vi "test3-SafeStr conversion.vi"(8 "error in (no error)":errorcluster, 11 "TestCase in":refnum<class "testcase-CSMArgument.lvclass">) -> (0 "error out":errorcluster, 3 "TestCase out":refnum<class "testcase-CSMArgument.lvclass">)   [LabVIEW 2017, in "testcase-CSMArgument.lvclass"]
uses:
  testcase-CSMArgument.lvclass
  src/user.lib/_NEVSTOP/Communicable State Machine(CSM)/AdvanceAPI/CSM - Keywords.vi
  <vilib>/addons/_JKI Toolkits/VI Tester/TestCase.llb/TestCase.lvclass
  src/user.lib/_NEVSTOP/Communicable State Machine(CSM)/Communicable State Machine.lvlib
  C:/Program Files (x86)/National Instruments/LabVIEW 2017/vi.lib/addons/_JKI Toolkits/VI Tester/TestCase.llb/TestCase.lvclass
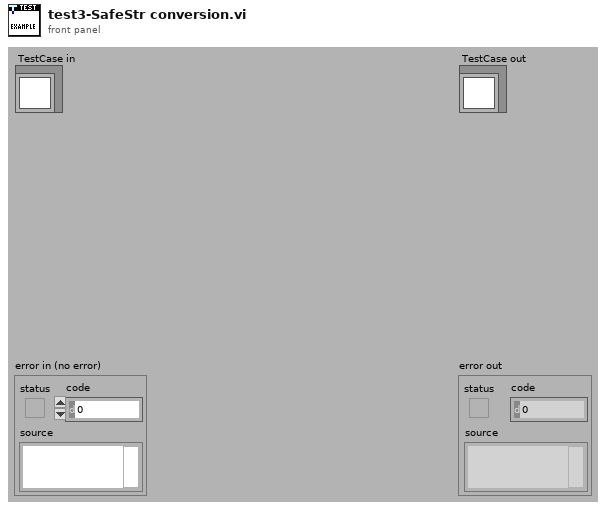
[diagram p1: front panel]
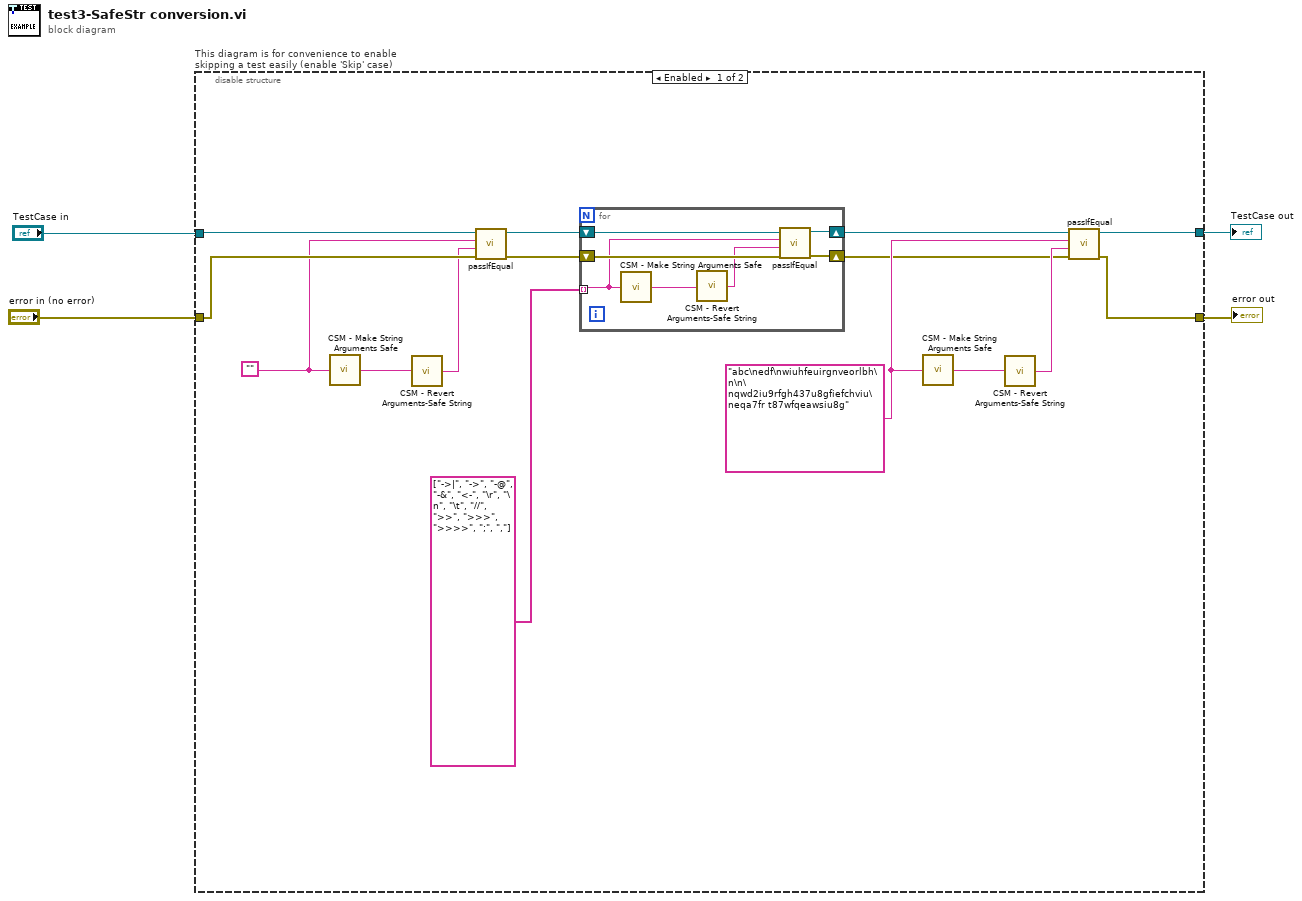
[diagram p0: block diagram]
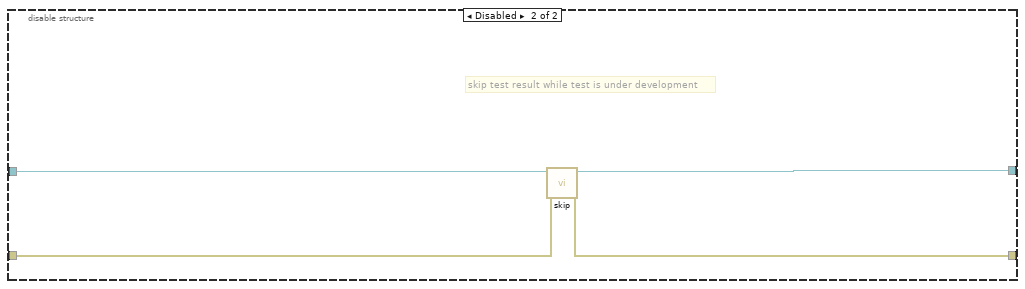
[diagram p2: hidden frame]
diagram:
  n1 = disable-structure "This diagram is for convenience to enable skipping a test easily (enable 'Skip' case)" shown="Enabled" {
    disable-tunnel: "TestCase in" -> [w19 w30]
    disable-tunnel: [w8 w28] -> w1
    disable-tunnel: [w6 w29] -> w3
    disable-tunnel: "error in (no error)" -> [w18 w27]
    frame Enabled {
      w10 = "abc\nedf\nwiuhfeuirgnveorlbh\n\n\nqwd2iu9rfgh437u8gfiefchviu\neqa7fr t87wfqeawsiu8g"
      w16 = ""
      n2 = call "CSM - Make String Arguments Safe.vi"("Argument String"=w16) -> ("Safe Argument String"=w17:string)  [unwired: 8 in]
      n3 = call "CSM - Revert Arguments-Safe String.vi"("Safe Argument String"=w17) -> ("Origin Argument String"=w15:string)  [unwired: 8 in]
      n4 = call-dynamic "passIfEqual.vi"("error in (no error)"=w18, "y"=w15, "x"=w16, "TestCase in"=w19) -> ("error out"=w12:errorcluster, "TestCase out"=w13:refnum<class "testcase-CSMArgument.lvclass">)  [unwired: 6 in]
      n5 = for {
        tunnel: string[] ["->|", "->", "-@", "-&", "<-", "\r", "\n", "\t", "//", ">>", ">>>", ">>>>", ";", ","] -> [w21] mode=indexing
        shift-right: [w24] -> w9
        shift-left: w13 -> [w25]
        shift-right: [w22] -> w7
        shift-left: w12 -> [w23]
        n6 = call "CSM - Make String Arguments Safe.vi"("Argument String"=w21) -> ("Safe Argument String"=w26:string)  [unwired: 8 in]
        n7 = call "CSM - Revert Arguments-Safe String.vi"("Safe Argument String"=w26) -> ("Origin Argument String"=w20:string)  [unwired: 8 in]
        n8 = call-dynamic "passIfEqual.vi"("error in (no error)"=w23, "y"=w20, "x"=w21, "TestCase in"=w25) -> ("error out"=w22:errorcluster, "TestCase out"=w24:refnum<class "testcase-CSMArgument.lvclass">)  [unwired: 6 in]
      }
      n9 = call "CSM - Make String Arguments Safe.vi"("Argument String"=w10) -> ("Safe Argument String"=w5:string)  [unwired: 8 in]
      n10 = call "CSM - Revert Arguments-Safe String.vi"("Safe Argument String"=w5) -> ("Origin Argument String"=w11:string)  [unwired: 8 in]
      n11 = call-dynamic "passIfEqual.vi"("error in (no error)"=w7, "y"=w11, "x"=w10, "TestCase in"=w9) -> ("error out"=w6:errorcluster, "TestCase out"=w8:refnum<class "testcase-CSMArgument.lvclass">)  [unwired: 6 in]
    }
    frame Disabled {
      # "skip test result while test is under development"
      n12 = call <vilib>:"skip.vi"("error in (no error)"=w27, "TestCase in"=w30) -> ("error out"=w29:errorcluster, "TestCase out"=w28:refnum<class "testcase-CSMArgument.lvclass">)  [unwired: 8 in]
    }
  }
  "error out" <- w3
  "TestCase out" <- w1
